vi "Time Stamp.vi"(5 "format string":string="%Y-%m-%dT%H:%M:%S%20u", 7 "key description":string, 8 "sections":string[](array[string]), 9 "time stamp":timestamp, 11 "info data":string) -> (0 "sections out":string[](array[string]), 3 "info data out":string)   [LabVIEW 2013, in "infolib.lvlib"]
doc: "Add a new date and time key to Info Data string. If section exists in Info Data string, inserts key into this section. If format is not set, ISO Date and Time format is used."
uses:
  infolib.lvlib
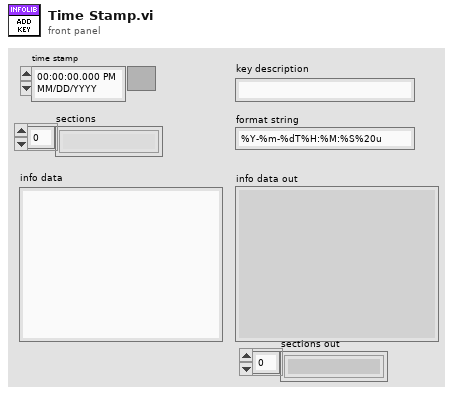
[diagram p1: front panel]
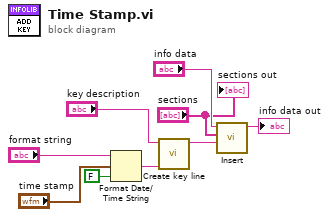
[diagram p0: block diagram]
diagram:
  n1 = Format Date/Time String(time format string (%c)="format string", seconds (now)="time stamp", UTC format=FALSE) -> (date/time string=w4:string)
  n2 = call "Create key line.vi"("formatted value"=w4, "key description"="key description") -> ("line"=w2:string)  [unwired: 9 in]
  n3 = call "Insert.vi"("insert"=w2, "sections"="sections", "info data"="info data") -> ("info data out"=→"info data out":string)  [unwired: 8 in]
  "sections out" <- "sections"
